vi "Snake Game.vi"() -> ()   [LabVIEW 2018]
uses:
  Typedefs/XYposition.ctl
  Typedefs/UnitDirection.ctl
  Typedefs/Colors.ctl
  Typedefs/DisplaySize.ctl
  LV_Classes/2D_Representer/2D_Representer.lvclass
panel:
  in  "Right":bool
  in  "Left":bool
  in  "Down":bool
  in  "Up":bool
  out "Snake":u32[][](array[colorbox])
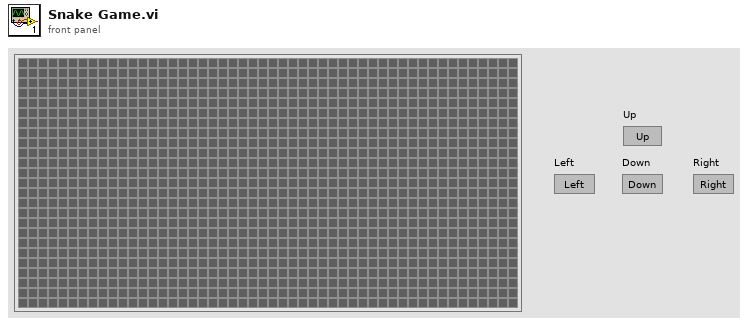
[diagram p1: front panel]
types:
  T1 = typedef "DisplaySize.ctl" = cluster{"Rows":i32, "Cols":i32}
  T2 = typedef "Colors.ctl" = cluster{"HeadColor":u32, "BodyColor":u32, "TailColor":u32, "FeedColor":u32}
  T3 = typedef "UnitDirection.ctl" = enum16{"North", "East", "South", "West"}
  T4 = typedef "XYposition.ctl" = cluster{"Col.LocX":i32, "Row.LocY":i32}
  T5 = typedef "eventvkey.ctl" = enum16{"ASCII", "Enter", "Return", "Shift", "Ctrl", "Alt", "Cmd", "Opt", "Caps", "NumLock", "Clear", "Break", "Up", "Down", "Left", "Right", "Insert", "Delete", "Home", "End", "PageUp", "PageDown", "Escape", "Help", "Pause", "ScrollLock", "F1", "F2", "F3", "F4", "F5", "F6", "F7", "F8", "F9", "F10", "F11", "F12", "F13", "F14", "F15", "F16", "F17", "F18", "F19", "F20", "F21", "F22", "F23", "F24", "Play", "VolumeUp", "VolumeDown", "Mute", "Two Byte Char"}
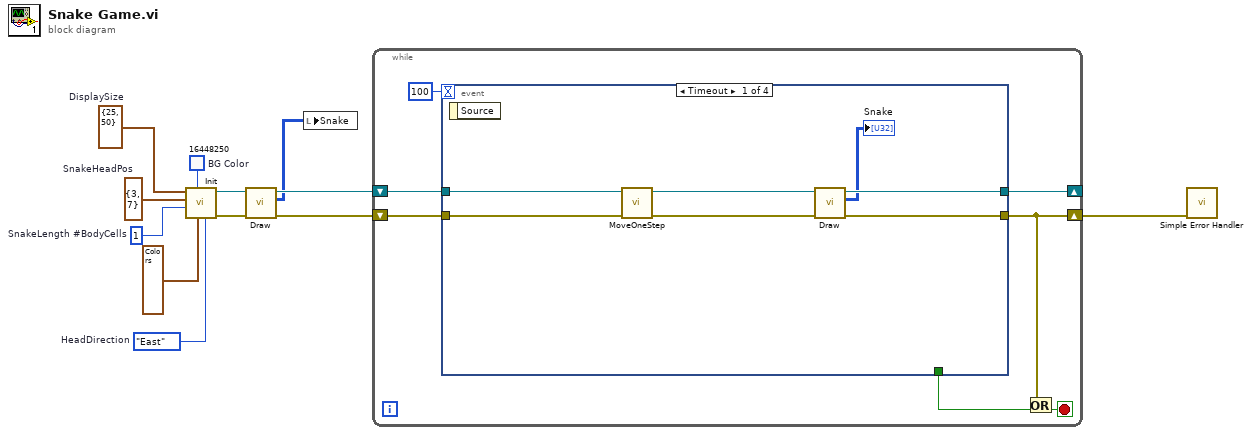
[diagram p0: block diagram]
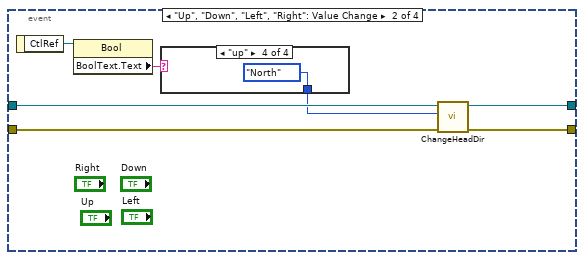
[diagram p2: hidden frame]
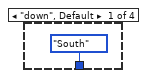
[diagram p3: hidden frame]
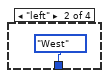
[diagram p4: hidden frame]
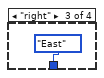
[diagram p5: hidden frame]
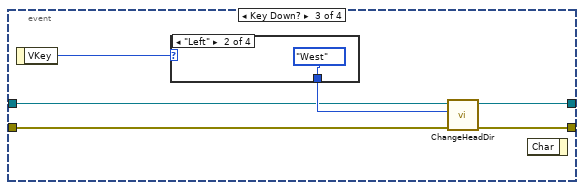
[diagram p6: hidden frame]
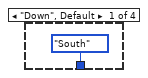
[diagram p7: hidden frame]
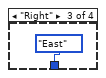
[diagram p8: hidden frame]
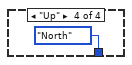
[diagram p9: hidden frame]
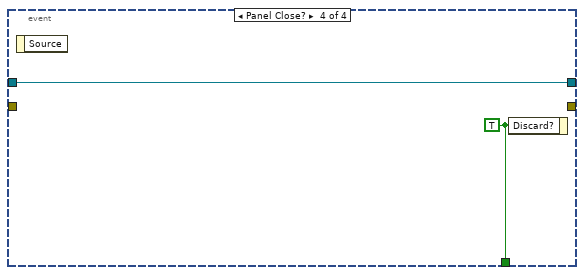
[diagram p10: hidden frame]
diagram:
  w7 = T1 {"Rows"=25, "Cols"=50}  # DisplaySize
  w9 = UnitDirection."East"  # HeadDirection
  w10 = u32 1  # SnakeLength #BodyCells
  w11 = T4 {"Col.LocX"=3, "Row.LocY"=7}  # SnakeHeadPos
  w12 = u32 16448250  # BG Color
  n1 = call "Init.vi"("HeadDirection"=w9, "SnakeColor"=T2 {"HeadColor"=16711680, "BodyColor"=32639, "TailColor"=7171459, "FeedColor"=16777224}, "BG Color"=w12, "SnakeLength #BodyCells"=w10, "SnakeHeadPos"=w11, "DisplaySize"=w7) -> ("error out"=w6:errorcluster, "2D_Representer out"=w3:refnum<class "2D_Representer.lvclass">)  [unwired: 4 in]
  n2 = call "Draw.vi"("error in (no error)"=w6, "2D_Representer in"=w3) -> ("error out"=w4:errorcluster, "Display Array"=w1:u32[][], "2D_Representer out"=w2:refnum<class "2D_Representer.lvclass">)  [unwired: 7 in]
  n3 = local write "Snake"(w1) -> ()
  n4 = while {
    shift-right: [w16] -> _
    shift-left: w2 -> [w17]
    shift-right: [w13] -> w5
    shift-left: w4 -> [w15]
    stop <- w14 stop-if-true
    n5 = event shown="[0] Timeout" {
      selector: _ -> [_ _ _ _]
      dyn-events: _ -> [_ _ _ _]
      timeout: 100 -> [_ _ _ _]
      tunnel: [_ _ _ w49] -> w18
      tunnel: w17 -> [w26 w31 w39 w48]
      tunnel: [w25 w30 w41 w48] -> w16
      tunnel: w15 -> [w22 w28 w38 _]
      tunnel: [w20 w27 w40 _] -> w13
      event Timeout {
        n6 = event-data() -> ()  [unwired: 1 in, 1 out]
        n7 = call "MoveOneStep.vi"("error in (no error)"=w22, "2D_Representer in"=w26) -> ("error out"=w21:errorcluster, "2D_Representer out"=w23:refnum<class "2D_Representer.lvclass">)  [unwired: 8 in]
        n8 = call "Draw.vi"("error in (no error)"=w21, "2D_Representer in"=w23) -> ("error out"=w20:errorcluster, "Display Array"=→"Snake":u32[][], "2D_Representer out"=w25:refnum<class "2D_Representer.lvclass">)  [unwired: 7 in]
      }
      event "Up", "Down", "Left", "Right": Value Change {
        n9 = event-data() -> ("CtlRef"=w33:refnum<vi>)  [unwired: 1 in]
        n10 = property class="Bool"(reference=w33) -> ("BoolText.Text"=w32:string)  [unwired: 1 in, 2 out]
        n11 = case shown="\"up\"" w32 {
          tunnel: [UnitDirection."South" ("UnitDirection") UnitDirection."West" ("UnitDirection") UnitDirection."East" ("UnitDirection") UnitDirection."North" ("UnitDirection")] -> w29
          frame "down", Default {
          }
          frame "left" {
          }
          frame "right" {
          }
          frame "up" {
          }
        }
        n12 = call "ChangeHeadDir.vi"("error in (no error)"=w28, "UnitDirection"=w29, "2D_Representer in"=w31) -> ("error out"=w27:errorcluster, "2D_Representer out"=w30:refnum<class "2D_Representer.lvclass">)  [unwired: 7 in]
      }
      event Key Down? {
        n13 = event-data() -> ("VKey"=w42:T5)  [unwired: 1 in]
        n14 = case shown="\"Left\"" w42 {
          tunnel: [UnitDirection."South" ("UnitDirection") UnitDirection."West" ("UnitDirection") UnitDirection."East" ("UnitDirection") UnitDirection."North" ("UnitDirection")] -> w43
          frame "Down", Default {
          }
          frame "Left" {
          }
          frame "Right" {
          }
          frame "Up" {
          }
        }
        n15 = call "ChangeHeadDir.vi"("error in (no error)"=w38, "UnitDirection"=w43, "2D_Representer in"=w39) -> ("error out"=w40:errorcluster, "2D_Representer out"=w41:refnum<class "2D_Representer.lvclass">)  [unwired: 7 in]
        n16 = event-data() -> ()  [unwired: 2 in, 1 out]
      }
      event Panel Close? {
        w49 = TRUE ("Discard?")
        n17 = event-data() -> ()  [unwired: 1 in, 1 out]
        n18 = event-data("Discard?"=w49) -> ()  [unwired: 1 in, 1 out]
      }
    }
    n19 = Or(x=w13, y=w18) -> (x .or. y?=w14:bool)
  }
  n20 = call <vilib>:"Simple Error Handler.vi"("error in (no error)"=w5) -> ()  [unwired: 4 in, 5 out]
